vi "CRYRestore Work State.vi"   [LabVIEW 2013]
uses:
  CRYHardware Global.vi
panel:
  # "Restore Hardware Work State"
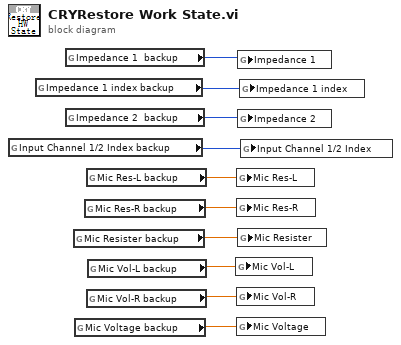
[diagram p0: block diagram]
diagram:
  n1 = global read "CRYHardware Global.vi" "Input Channel 1/2 Index backup"() -> (w4:i32)
  n2 = global read "CRYHardware Global.vi" "Impedance 1 index backup"() -> (w2:i32)
  n3 = global read "CRYHardware Global.vi" "Impedance 1  backup"() -> (w1:i32)
  n4 = global read "CRYHardware Global.vi" "Impedance 2  backup"() -> (w3:i32)
  n5 = global read "CRYHardware Global.vi" "Mic Resister backup"() -> (w7:dbl)
  n6 = global read "CRYHardware Global.vi" "Mic Voltage backup"() -> (w10:dbl)
  n7 = global read "CRYHardware Global.vi" "Mic Res-R backup"() -> (w6:dbl)
  n8 = global read "CRYHardware Global.vi" "Mic Res-L backup"() -> (w5:dbl)
  n9 = global read "CRYHardware Global.vi" "Mic Vol-R backup"() -> (w9:dbl)
  n10 = global read "CRYHardware Global.vi" "Mic Vol-L backup"() -> (w8:dbl)
  n11 = global write "CRYHardware Global.vi" "Mic Vol-L"(w8) -> ()
  n12 = global write "CRYHardware Global.vi" "Mic Res-L"(w5) -> ()
  n13 = global write "CRYHardware Global.vi" "Mic Res-R"(w6) -> ()
  n14 = global write "CRYHardware Global.vi" "Mic Vol-R"(w9) -> ()
  n15 = global write "CRYHardware Global.vi" "Mic Voltage"(w10) -> ()
  n16 = global write "CRYHardware Global.vi" "Impedance 1"(w1) -> ()
  n17 = global write "CRYHardware Global.vi" "Impedance 2"(w3) -> ()
  n18 = global write "CRYHardware Global.vi" "Mic Resister"(w7) -> ()
  n19 = global write "CRYHardware Global.vi" "Impedance 1 index"(w2) -> ()
  n20 = global write "CRYHardware Global.vi" "Input Channel 1/2 Index"(w4) -> ()
